vi "PKG_IMC_ArcLine_Dist.vi"(0 "handle":u32, 1 "dist_x":i32, 2 "dist_y":i32, 3 "dist_cx":i32, 4 "dist_cy":i32, 5 "dir":i32, 6 "dist":i32[](array[numeric])=array[4097 elements], 8 "axisNum":i32, 9 "tgvel":dbl, 10 "endvel":dbl, 11 "wait":i32, 12 "fifo":i32) -> (20 "handle out":u32, 21 "function return":i32, 26 "dist out":i32[](array[numeric]))   [LabVIEW 2011, in "IMC_Pkg4xxx.lvlib"]
doc: "PKG_IMC_ArcLine_Dist(IMC_HANDLE handle, long dist_x, long dist_y, long dist_cx, long dist_cy, int dir, long dist[], int axisNum, double tgvel, double endvel, int wait, int fifo);"
uses:
  IMC_Pkg4xxx.lvlib
  IMC_Pkg4xxx.dll
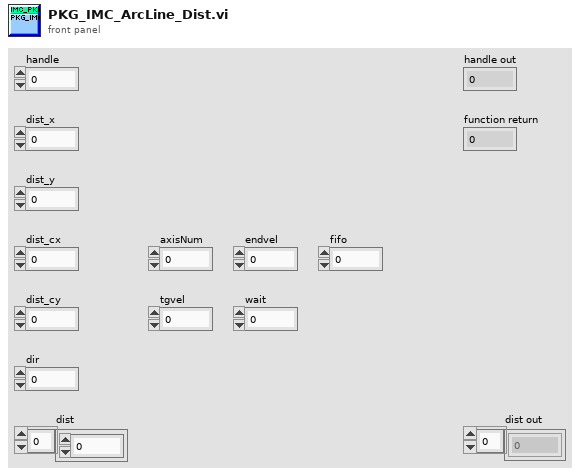
[diagram p1: front panel]
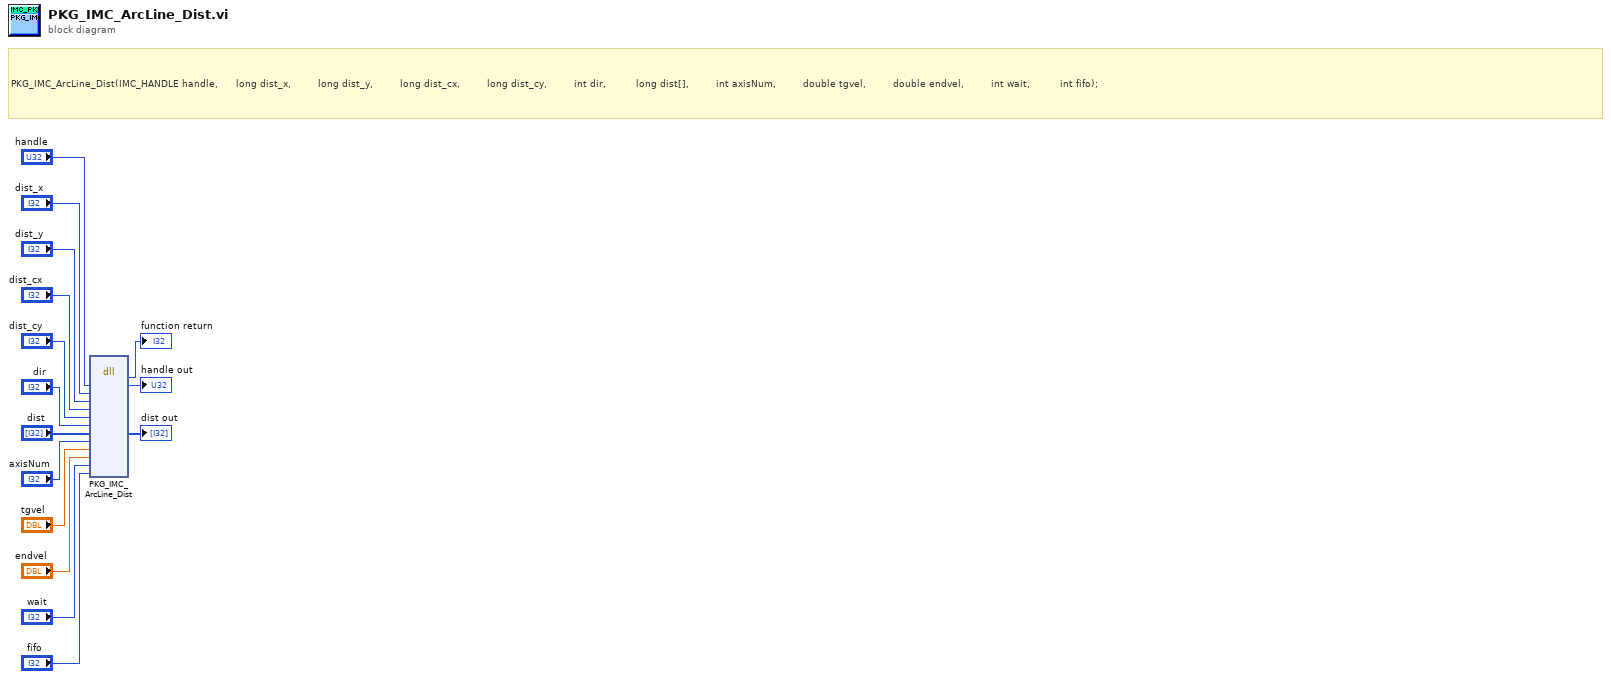
[diagram p0: block diagram]
diagram:
  # "PKG_IMC_ArcLine_Dist(IMC_HANDLE handle, \t\t\t\t\tlong dist_x, \t\t\t\t\t\t\t\tlong dist_y, \t\t\t\t\t\t\t\tlong dist_cx, \t\t\t\t\t\t\t\tlong dist_cy, \t\t\t\t\t\t\t\tint dir, \t\t\t\t\t\t\t\t\tlong dist[], \t\t\t\t\t\t\t\tint axisNum, \t\t\t\t\t\t\t\tdouble tgvel, \t\t\t\t\t\t\t\tdouble endvel, \t\t\t\t\t\t\t\tint wait, \t\t\t\t\t\t\t\t\tint fifo);"
  n1 = dll-call lib="PTH1mabs F光盘刻录\niMC MotionIMCNet_V4.0IMCAppincLabviewIMC_PKG4xxxIMC_PKG4xxx\nIMC_Pkg4xxx.*" fn="PKG_IMC_ArcLine_Dist"("handle"="handle", "dist_x"="dist_x", "dist_y"="dist_y", "dist_cx"="dist_cx", "dist_cy"="dist_cy", "dir"="dir", "dist"="dist", "axisNum"="axisNum", "tgvel"="tgvel", "endvel"="endvel", "wait"="wait", "fifo"="fifo") -> (→"function return":i32, "handle"=→"handle out":u32, "dist"=→"dist out":i32[])  [unwired: 13 in, 2 out]
